vi "Load_All_Transconductance_2D angles_use this one.vi"() -> ()   [LabVIEW 2016]
panel:
  out "peak diff large":T1(graph)
  out "large angles":dbl[][](array[numeric])
  out "peak diff small":T1(graph)
  out "Intensity Graph 15":dbl[][](graph)
  in  "index (page)":i32=3
  out "Intensity Graph 14":dbl[][](graph)
  out "small angles":dbl[][](array[numeric])
  in  "read data from file?":bool
  out "All Folders":path[](array[path])=[path "P:/expt/Leiden MNK/SA02836H.20170110/40/40 - Sweep axis 1,2 - 0", path "P:/expt/Leiden MNK/SA02836H.20170110/40/40 - Sweep axis 1,2 - 1", path "P:/expt/Leiden MNK/SA02836H.20170110/40/40 - Sweep axis 1,2 - 2", path "P:/expt/Leiden MNK/SA02836H.20170110/40/40 - Sweep axis 1,2 - 3", path "P:/expt/Leiden MNK/SA02836H.20170110/40/40 - Sweep axis 1,2 - 4", path "P:/expt/Leiden MNK/SA02836H.20170110/40/40 - Sweep axis 1,2 - 5", path "P:/expt/Leiden MNK/SA02836H.20170110/40/40 - Sweep axis 1,2 - 6", path "P:/expt/Leiden MNK/SA02836H.20170110/40/40 - Sweep axis 1,2 - 7", path "P:/expt/Leiden MNK/SA02836H.20170110/40/40 - Sweep axis 1,2 - 8", path "P:/expt/Leiden MNK/SA02836H.20170110/40/40 - Sweep axis 1,2 - 9", path "P:/expt/Leiden MNK/SA02836H.20170110/40/x40 - Sweep axis 1,2 - 10"]
  out "Numeric":i32=10
  out "Array":i32[][](array[numeric])
  in  "Array 2":path[](array[path])=[path "P:/expt/Leiden MNK/SA02836H.20170110/40"]
  out "Intensity Graph 12":dbl[][][](array[numeric])
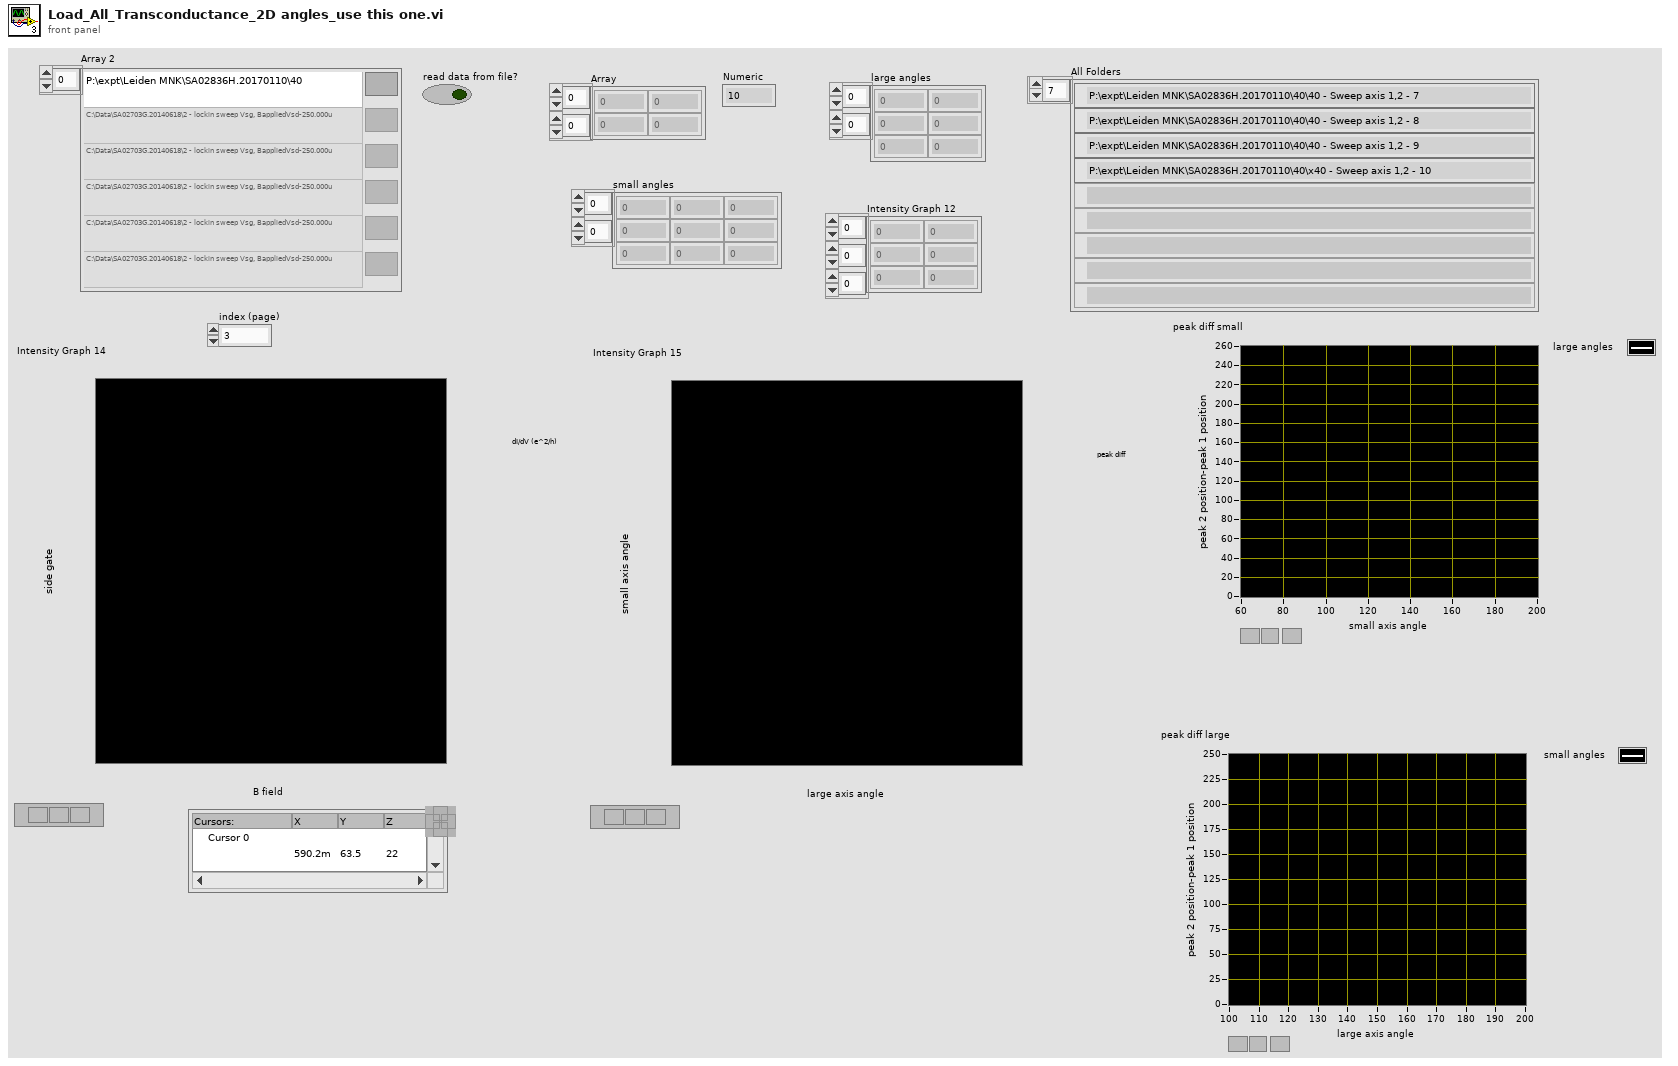
[diagram p1: front panel]
types:
  T1 = cluster{"Vfast":dbl[], "Decimated Array":dbl[]}[]
  T2 = cluster{"N1":dbl, "N2":dbl, "N3":dbl, "N4":dbl}[]
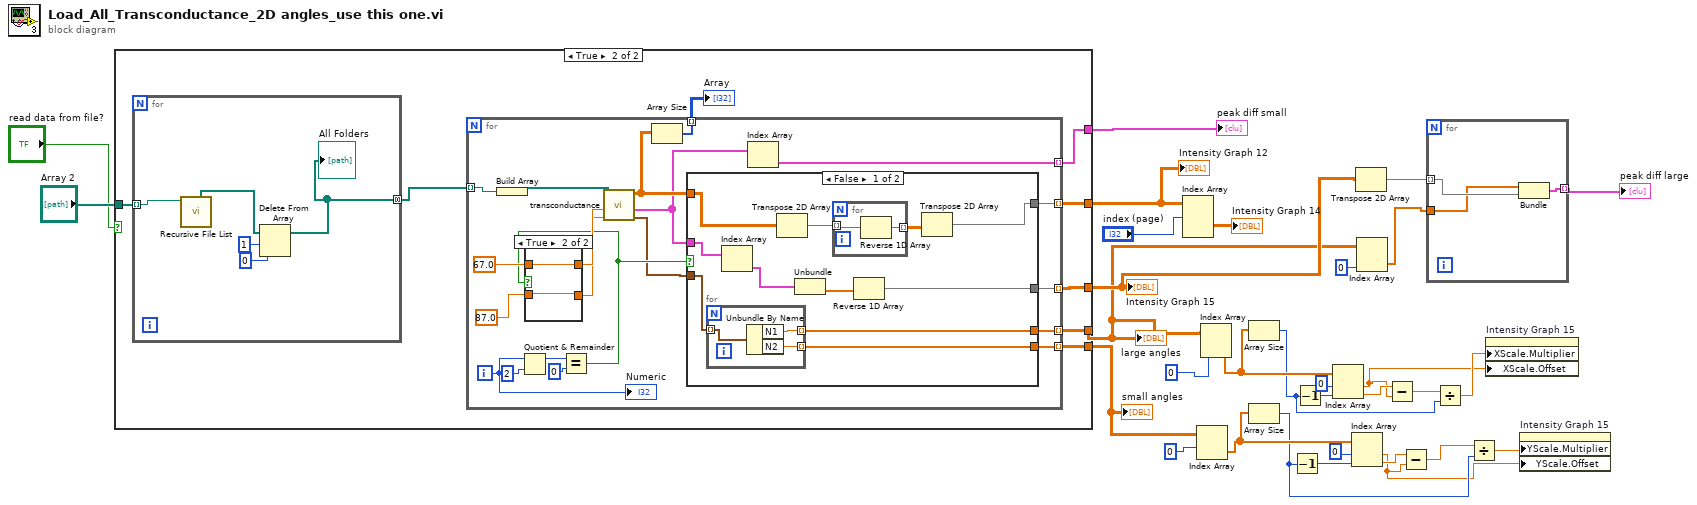
[diagram p0: block diagram]
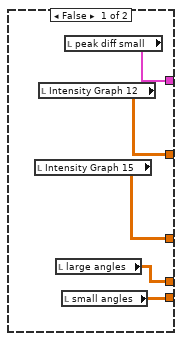
[diagram p2: hidden frame]
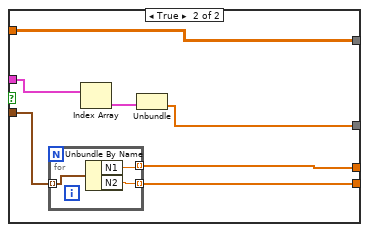
[diagram p3: hidden frame]
diagram:
  n1 = case shown="True" "read data from file?" {
    tunnel: "Array 2" -> [_ w44]
    tunnel: [w36 w42] -> w28
    tunnel: [w35 w40] -> w25
    tunnel: [w34 w39] -> w5
    tunnel: [w33 w38] -> w26
    tunnel: [w32 w37] -> w1
    frame False {
      n2 = local read "Intensity Graph 15"() -> (w34:dbl[][])
      n3 = local read "Intensity Graph 12"() -> (w36:dbl[][][])
      n4 = local read "large angles"() -> (w32:dbl[][])
      n5 = local read "small angles"() -> (w35:dbl[][])
      n6 = local read "peak diff small"() -> (w33:T1)
    }
    frame True {
      n7 = for {
        tunnel: w44 -> [w99] mode=indexing
        tunnel: [w95] -> w43 mode=concatenating
        n8 = call <vilib>:"Recursive File List.vi"("Folder Path"=w99) -> ("All Folders"=w98:path[])  [unwired: 6 in, 4 out]
        n9 = Delete From Array(array=w98, length=1, index=0) -> (array with subset deleted=w95:path[])  [unwired: 1 out]
        "All Folders" <- w95
      }
      n10 = for {
        tunnel: w43 -> [w64] mode=indexing
        tunnel: [w58] -> w42 mode=indexing
        tunnel: [w51] -> w41 mode=indexing
        tunnel: [w49] -> w40 mode=indexing
        tunnel: [w45] -> w39 mode=indexing
        tunnel: [w48] -> w38 mode=indexing
        tunnel: [w47] -> w37 mode=indexing
        i -> [w57]
        n11 = Build Array(w64) -> (w63:path[])
        n12 = Quotient & Remainder(x=w57, y=2) -> (x-y*floor(x/y)=w55:i32)  [unwired: 1 out]
        n13 = Equal?(x=w55, y=0) -> (x = y?=w53:bool)
        n14 = call "transconductance.vi"("New Files to Process"=w63) -> ("N Array"=w50:T2, "peak diff"=w46:T1, "Intensity Graph 12"=w52:dbl[][], "B max"=w59:dbl, "B min"=w61:dbl)  [unwired: 5 in, 1 out]
        n15 = case shown="True" w53 {
          tunnel: 67.0 ("B min") -> [w91 w94]
          tunnel: w61 -> [w92 w94]
          tunnel: 87.0 ("B max") -> [w92 w93]
          tunnel: w59 -> [w91 w93]
          frame False {
          }
          frame True {
          }
        }
        n16 = Array Size(array=w52) -> (size(s)=w51:i32[])
        n17 = case shown="False" w53 {
          tunnel: w52 -> [w75 w87]
          tunnel: [w72 w87] -> w58
          tunnel: w50 -> [w71 w86]
          tunnel: [w70 w85] -> w49
          tunnel: [w69 w84] -> w47
          tunnel: w46 -> [w68 w83]
          tunnel: [w65 w81] -> w45
          frame False {
            n18 = for {
              tunnel: w71 -> [w78] mode=indexing
              tunnel: [w77] -> w69 mode=indexing
              tunnel: [w76] -> w70 mode=indexing
              n19 = Unbundle By Name(w78) -> ("N1"=w77:dbl, "N2"=w76:dbl)
            }
            n20 = Index Array(array=w68) -> (element=w67:cluster{"Vfast":dbl[], "Decimated Array":dbl[]})  [unwired: 1 in]
            n21 = Transpose 2D Array(2D array=w75) -> (transposed array=w74:dbl[][])
            n22 = Unbundle(w67) -> ("Decimated Array"=w66:dbl[])  [unwired: 1 out]
            n23 = for {
              tunnel: w74 -> [w80] mode=indexing
              tunnel: [w79] -> w73 mode=indexing
              n24 = Reverse 1D Array(array=w80) -> (reversed array=w79:dbl[])
            }
            n25 = Reverse 1D Array(array=w66) -> (reversed array=w65:dbl[])
            n26 = Transpose 2D Array(2D array=w73) -> (transposed array=w72:dbl[][])
          }
          frame True {
            n27 = for {
              tunnel: w86 -> [w90] mode=indexing
              tunnel: [w89] -> w85 mode=indexing
              tunnel: [w88] -> w84 mode=indexing
              n28 = Unbundle By Name(w90) -> ("N1"=w88:dbl, "N2"=w89:dbl)
            }
            n29 = Index Array(array=w83) -> (element=w82:cluster{"Vfast":dbl[], "Decimated Array":dbl[]})  [unwired: 1 in]
            n30 = Unbundle(w82) -> ("Decimated Array"=w81:dbl[])  [unwired: 1 out]
          }
        }
        n31 = Index Array(array=w46) -> (element=w48:cluster{"Vfast":dbl[], "Decimated Array":dbl[]})  [unwired: 1 in]
        "Numeric" <- w57
      }
      "Array" <- w41
    }
  }
  "Intensity Graph 12" <- w28
  "small angles" <- w25
  "Intensity Graph 15" <- w5
  "peak diff small" <- w26
  "large angles" <- w1
  n32 = Index Array(array=w28, index (dim 0)="index (page)") -> (element=→"Intensity Graph 14":dbl[][])  [unwired: 2 in]
  n33 = Index Array(array=w25, index (row)=0) -> (element=w20:dbl[])  [unwired: 1 in]
  n34 = Index Array(array=w1, index (col)=0 ("index (row)")) -> (element=w22:dbl[])  [unwired: 1 in]
  n35 = Array Size(array=w22) -> (size(s)=w16:i32)
  n36 = Array Size(array=w20) -> (size(s)=w15:i32)
  n37 = Decrement(x=w15) -> (x-1=w19:i32)
  n38 = Decrement(x=w16) -> (x-1=w17:i32)
  n39 = Index Array(array=w22, index #1=0 ("index (row)"), index #2=w17) -> (element #1=w7:dbl, element #2=w8:dbl)
  n40 = Index Array(array=w20, index #1=0 ("index (row)"), index #2=w19) -> (element #1=w9:dbl, element #2=w10:dbl)
  n41 = Transpose 2D Array(2D array=w5) -> (transposed array=w6:dbl[][])
  n42 = Index Array(array=w1, index (col)=0 ("disabled index (col)")) -> (element=w3:dbl[])  [unwired: 1 in]
  n43 = Subtract(x=w8, y=w7) -> (x-y=w12:dbl)
  n44 = Subtract(x=w10, y=w9) -> (x-y=w11:dbl)
  n45 = for {
    tunnel: w6 -> [w101] mode=indexing
    tunnel: w3 -> [w100]
    tunnel: [w102] -> w2 mode=indexing
    n46 = Bundle("large angles"=w100, w101) -> (w102:cluster{"large angles":dbl[], dbl[]})  [unwired: 1 in]
  }
  "peak diff large" <- w2
  n47 = Divide(x=w12, y=w16) -> (x/y=w13:dbl)
  n48 = Divide(x=w11, y=w15) -> (x/y=w14:dbl)
  n49 = property on="Intensity Graph 15" class="IntGraph (strict)"("XScale.Multiplier"=w13, "XScale.Offset"=w7) -> ()  [unwired: 2 in, 2 out]
  n50 = property on="Intensity Graph 15" class="IntGraph (strict)"("YScale.Multiplier"=w14, "YScale.Offset"=w9) -> ()  [unwired: 2 in, 2 out]
